vi "Com Par.vi"(8 "error in (no error)":errorcluster) -> (0 "error out":errorcluster)   [LabVIEW 2014]
uses:
  <vilib>/Instr/_visa.llb/VISA Find Search Mode.ctl
  Controls/Global.vi
panel:
  out "取消":bool
  out "保存":bool
  in  "数据位":u16(ring) items=["5"=5, "6"=6, "7"=7, "8"=8]
  in  "停止位":u16(ring) items=["1"=10, "1.5"=15, "2"=20]
  in  "波特率":u16(ring) items=["9600"=9600, "56000"=56000, "115200"=2]
  in  "串口":u16(ring) items=["COM3"]
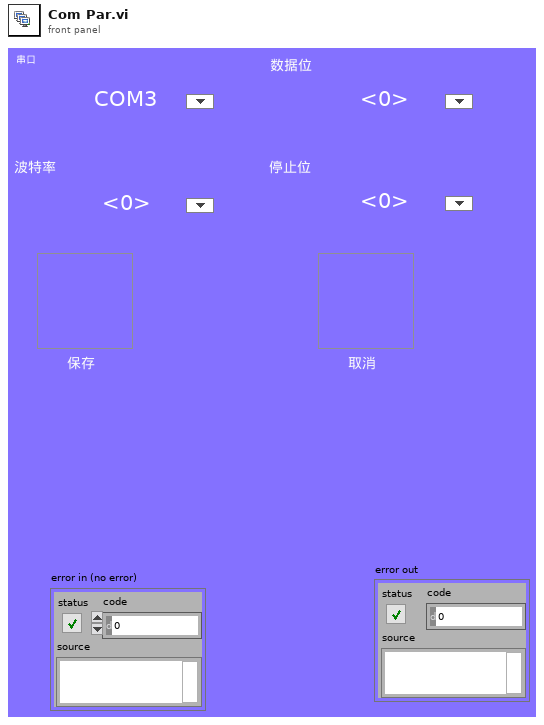
[diagram p1: front panel]
types:
  T1 = enum16{"Initialize", "Log", "Delete", "Stop", "Idle"}
  T2 = typedef "VISA Find Search Mode.ctl" = u32
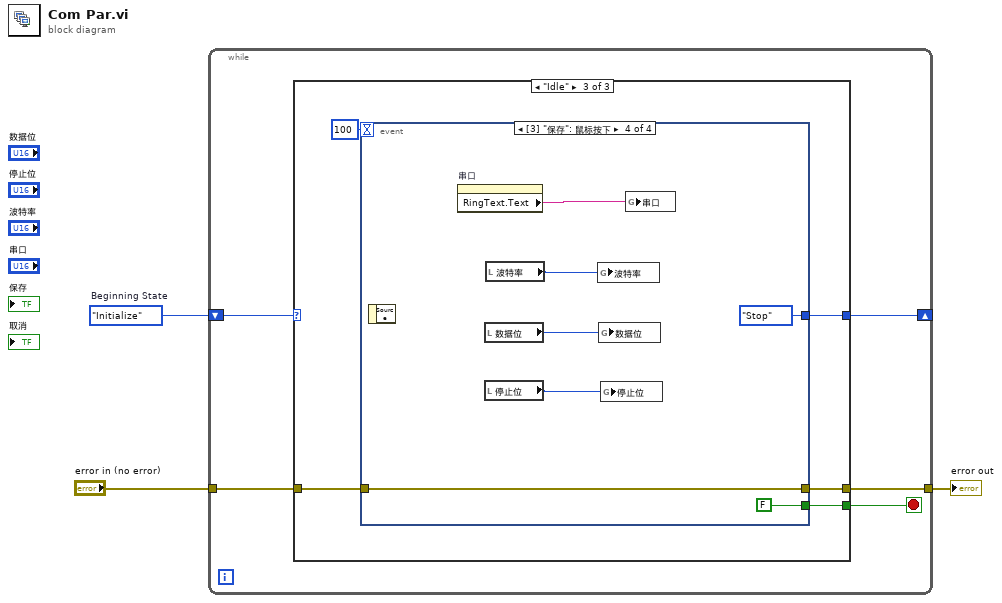
[diagram p0: block diagram]
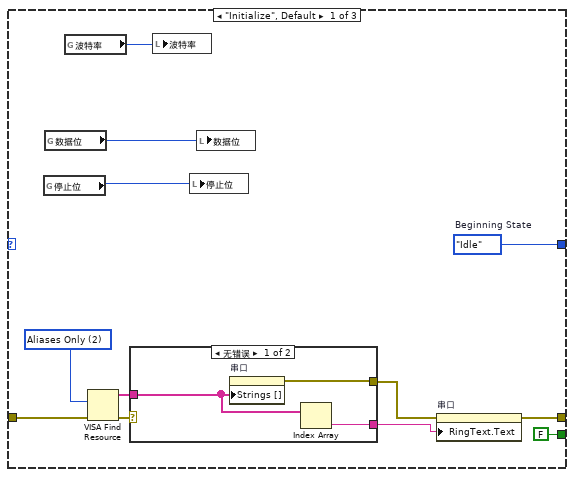
[diagram p2: hidden frame]
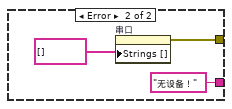
[diagram p3: hidden frame]
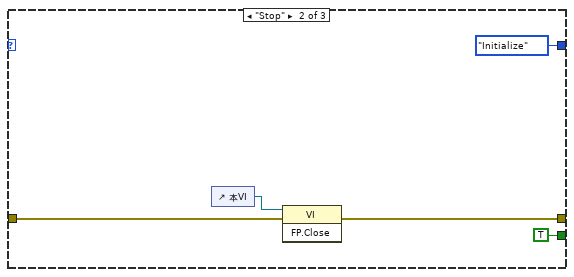
[diagram p4: hidden frame]
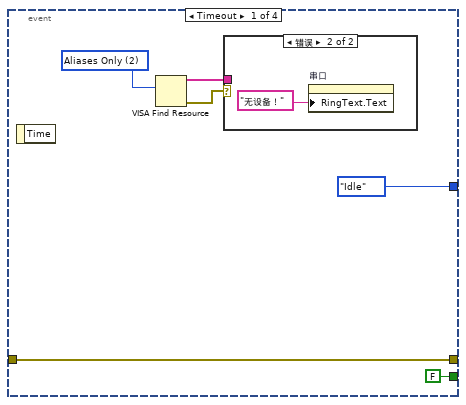
[diagram p5: hidden frame]
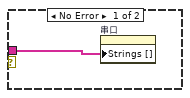
[diagram p6: hidden frame]
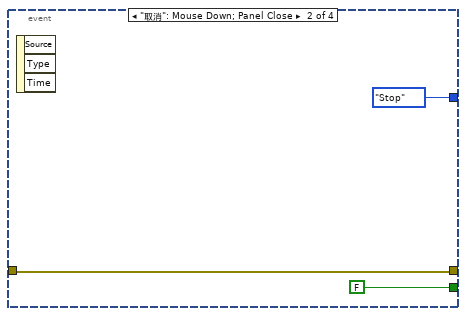
[diagram p7: hidden frame]
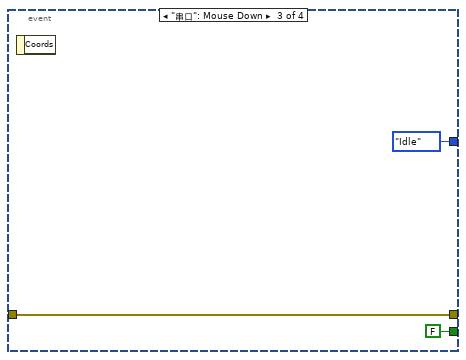
[diagram p8: hidden frame]
diagram:
  w1 = T1."Initialize"  # Beginning State
  n1 = while {
    tunnel: "error in (no error)" -> [w7]
    tunnel: [w6] -> w2
    shift-right: [w4] -> _
    shift-left: w1 -> [w5]
    stop <- w8 stop-if-true
    n2 = case shown="\"Idle\"" w5 {
      tunnel: [FALSE TRUE w35] -> w8
      tunnel: w7 -> [w17 w31 w34]
      tunnel: [w15 w30 w33] -> w6
      tunnel: [w19 T1."Initialize" ("Beginning State") w32] -> w4
      frame "Initialize", Default {
        w18 = T2 2 items=["Canonical Names Only"=0, "Aliases Only"=2, "Include Matching Aliases"=3, "Include All Aliases"=4] ("Search Mode")
        w19 = T1."Idle"  # Beginning State
        n3 = global read "Global.vi" "停止位"() -> (w9:u16)
        n4 = global read "Global.vi" "数据位"() -> (w11:u16)
        n5 = global read "Global.vi" "波特率"() -> (w10:u32)
        n6 = VISA Find Resource(8:w17, 10:w18) -> (0:w16:errorcluster, 3:w14:string[])  [unwired: 1 in, 1 out]
        n7 = case shown="无错误" w16 {
          tunnel: w14 -> [w22 _]
          tunnel: [w23 w25] -> w13
          tunnel: [w21 "无设备！"] -> w12
          frame No Error {
            n8 = property on="串口" class="Ring (严格)"("Strings []"=w22) -> (error out=w23:errorcluster)  [unwired: 2 in, 1 out]
            n9 = Index Array(array=w22) -> (element=w21:string)  [unwired: 1 in]
          }
          frame Error {
            n10 = property on="串口" class="Ring (严格)"("Strings []"=string[] []) -> (error out=w25:errorcluster)  [unwired: 2 in, 1 out]
          }
        }
        n11 = local write "波特率"(w10) -> ()
        n12 = local write "停止位"(w9) -> ()
        n13 = local write "数据位"(w11) -> ()
        n14 = property on="串口" class="Ring (严格)"(error in=w13, "RingText.Text"=w12) -> (error out=w15:errorcluster)  [unwired: 1 in, 1 out]
      }
      frame "Stop" {
        n15 = control-ref of="本VI"() -> (w27:refnum<vi>)
        n16 = invoke class="VI" method="FP.Close"(reference=w27, error in=w31) -> (error out=w30:errorcluster)  [unwired: 1 in, 2 out]
      }
      frame "Idle" {
        n17 = event shown="[3] \"保存\": 鼠标按下" {
          selector: _ -> [_ _ _ _]
          dyn-events: _ -> [_ _ _ _]
          timeout: 100 -> [_ _ _ _]
          tunnel: [FALSE FALSE FALSE FALSE] -> w35
          tunnel: w34 -> [w40 w45 w49 w56]
          tunnel: [w40 w45 w49 w56] -> w33
          tunnel: [T1."Idle" ("Beginning State") T1."Stop" ("Beginning State") T1."Idle" ("Beginning State") T1."Stop" ("Beginning State")] -> w32
          event Timeout {
            w39 = T2 2 items=["Canonical Names Only"=0, "Aliases Only"=2, "Include Matching Aliases"=3, "Include All Aliases"=4] ("Search Mode")
            n18 = event-data() -> ()  [unwired: 1 in, 1 out]
            n19 = VISA Find Resource(10:w39) -> (0:w38:errorcluster, 3:w37:string[])  [unwired: 2 in, 1 out]
            n20 = case shown="错误" w38 {
              tunnel: w37 -> [w43 _]
              frame No Error {
                n21 = property on="串口" class="Ring (严格)"("Strings []"=w43) -> ()  [unwired: 2 in, 2 out]
              }
              frame Error {
                n22 = property on="串口" class="Ring (严格)"("RingText.Text"="无设备！" ("Ring Text.Text")) -> ()  [unwired: 2 in, 2 out]
              }
            }
          }
          event "取消": Mouse Down; Panel Close {
            n23 = event-data() -> ()  [unwired: 1 in, 3 out]
          }
          event "串口": Mouse Down {
            n24 = event-data() -> ()  [unwired: 1 in, 1 out]
          }
          event "保存": Mouse Down {
            n25 = event-data() -> ()  [unwired: 1 in, 1 out]
            n26 = property on="串口" class="Ring (严格)"() -> ("RingText.Text"=w57:string)  [unwired: 2 in, 2 out]
            n27 = local read "数据位"() -> (w51:u16)
            n28 = local read "停止位"() -> (w52:u16)
            n29 = local read "波特率"() -> (w53:u16)
            n30 = global write "Global.vi" "波特率"(w53) -> ()
            n31 = global write "Global.vi" "数据位"(w51) -> ()
            n32 = global write "Global.vi" "停止位"(w52) -> ()
            n33 = global write "Global.vi" "串口"(w57) -> ()
          }
        }
      }
    }
  }
  "error out" <- w2
